vi "asset.free.vi"(8 "error in":errorcluster, 11 "object_in":refnum<class "Asset.lvclass">) -> (0 "error out":errorcluster, 3 "object_out":refnum<class "Asset.lvclass">)   [LabVIEW 2020, in "Asset.lvclass"]
doc: "Releases the handle and its associated resources."
uses:
  Asset.lvclass
  Asset.lvclass/Asset.ctl
  client.lvlib
panel:
  out "function return":i32
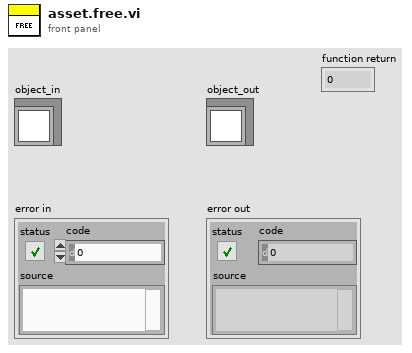
[diagram p1: front panel]
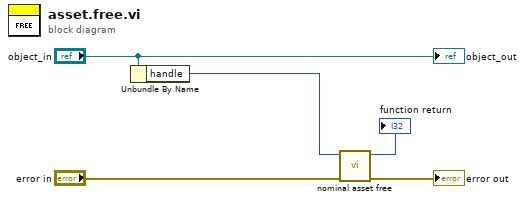
[diagram p0: block diagram]
diagram:
  n1 = Unbundle By Name("object_in") -> ("handle"=w3:i32)
  n2 = call "nominal asset free.vi"("error in (no error)"="error in", "asset"=w3) -> ("error out"=→"error out":errorcluster, "function return"=→"function return":i32)  [unwired: 8 in]
  "object_out" <- "object_in"
